vi "Global_SM_Data Out.vi"() -> ()   [LabVIEW 2017, in "Hopper System.lvlib"]
uses:
  Hopper System.lvlib
panel:
  in  "CMD_Hopper Feed":dbl
  out "Hopper_SM_Shooting Complete":bool
  in  "Hopper_SM_Inner Speed":dbl
  in  "Hopper_SM_Loader Speed":dbl
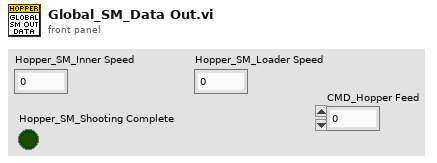
[diagram p1: front panel]
diagram:
